vi "get engine reference.vi"(8 "error in":errorcluster, 11 "engine mappings":refnum<data-value>) -> (0 "error out":errorcluster, 3 "engine reference":refnum<data-value>)   [LabVIEW 2013, in "PL Framework Configuration Tool.lvlib" / "Engine Mappings.lvclass"]
uses:
  Engine Mappings.lvclass
  Engine Parent/Engine Parent Editor Node.lvclass
  <vilib>/NI/Configuration Framework/Node/NISE_CEF_Node.lvclass/NISE_CEF_Node.ctl
  <vilib>/NI/Configuration Framework/Node/ReadParent.vi
  <vilib>/NI/Configuration Framework/Node/NISE_CEF_Node.lvclass
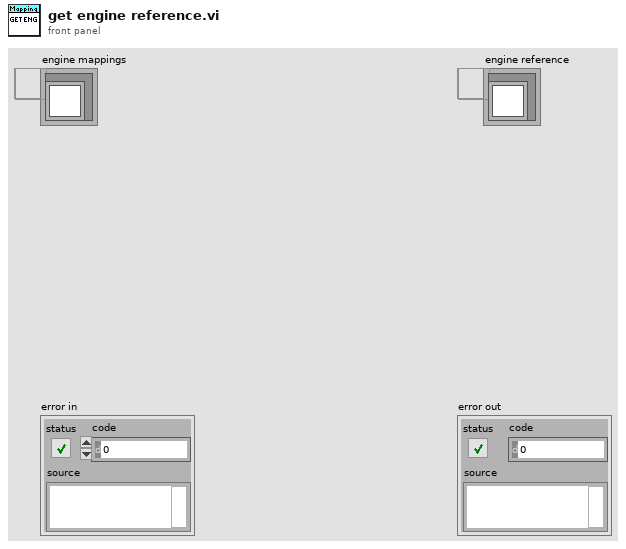
[diagram p1: front panel]
types:
  T1 = typedef "NISE_CEF_Node.lvclass/NodeRef.ctl" = refnum<data-value>
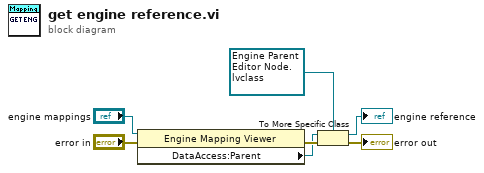
[diagram p0: block diagram]
diagram:
  n1 = property class="Engine Mapping Viewer"(reference="engine mappings", error in="error in") -> (error out=w7:errorcluster, "DataAccess:Parent"=w6:T1)  [unwired: 1 out]
  n2 = To More Specific Class(target class=refnum<data-value> refnum ("engine reference"), reference=w6, error in=w7) -> (specific class reference=→"engine reference":refnum<data-value>, error out=→"error out":errorcluster)
